vi "ConvertBoolArray4x8ToIntArray1x32.vi"(7 "boolMatrix4x8":bool[][](array[boolean])) -> (8 "intArray1x32":u32[](array[numeric]))   [LabVIEW 2016]
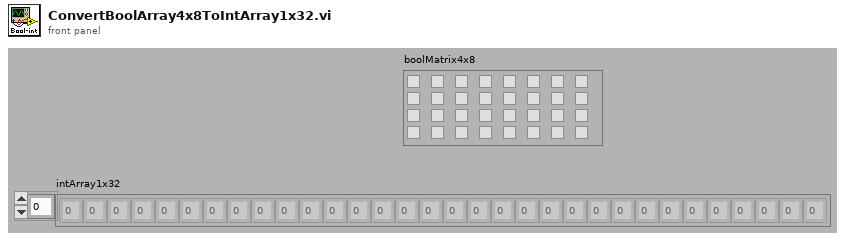
[diagram p1: front panel]
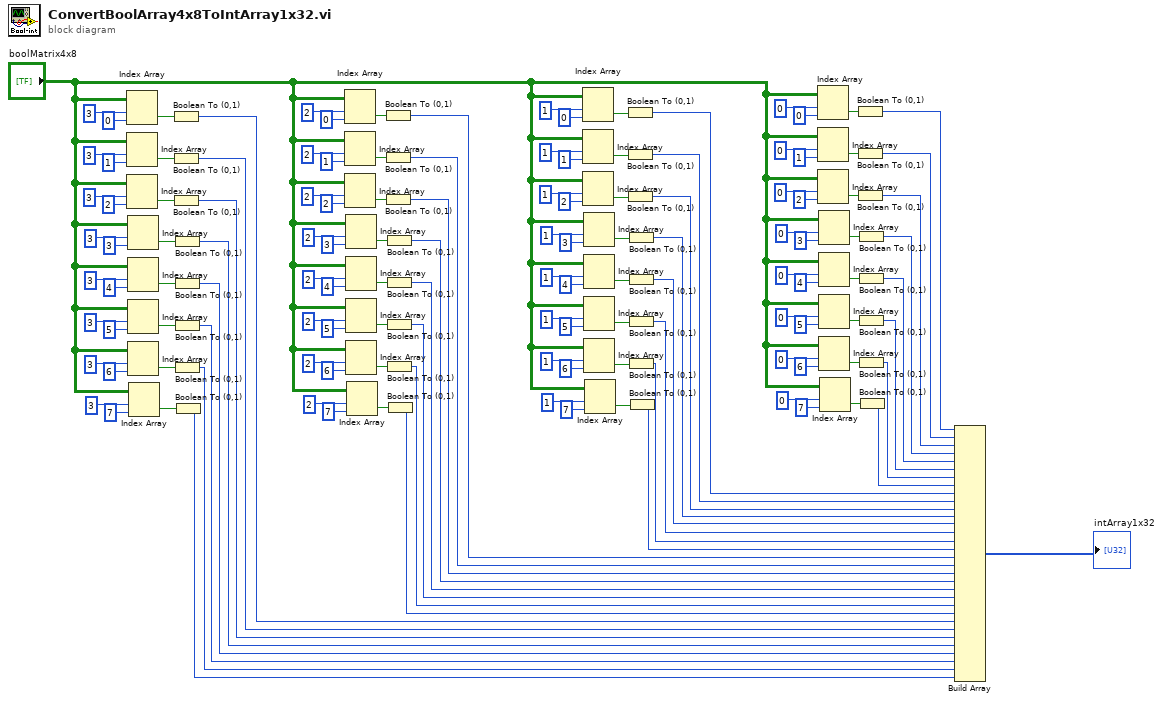
[diagram p0: block diagram]
diagram:
  n1 = Index Array(array="boolMatrix4x8", index (row)=3, index (col)=0) -> (element=w10:bool)
  n2 = Index Array(array="boolMatrix4x8", index (row)=3, index (col)=1) -> (element=w11:bool)
  n3 = Index Array(array="boolMatrix4x8", index (row)=3, index (col)=2) -> (element=w12:bool)
  n4 = Index Array(array="boolMatrix4x8", index (row)=3, index (col)=3) -> (element=w13:bool)
  n5 = Index Array(array="boolMatrix4x8", index (row)=3, index (col)=4) -> (element=w14:bool)
  n6 = Index Array(array="boolMatrix4x8", index (row)=3, index (col)=5) -> (element=w15:bool)
  n7 = Index Array(array="boolMatrix4x8", index (row)=3, index (col)=6) -> (element=w16:bool)
  n8 = Index Array(array="boolMatrix4x8", index (row)=3, index (col)=7) -> (element=w17:bool)
  n9 = Boolean To (0,1)(Boolean=w10) -> (0, 1=w9:i16)
  n10 = Boolean To (0,1)(Boolean=w11) -> (0, 1=w8:i16)
  n11 = Boolean To (0,1)(Boolean=w12) -> (0, 1=w7:i16)
  n12 = Boolean To (0,1)(Boolean=w13) -> (0, 1=w6:i16)
  n13 = Boolean To (0,1)(Boolean=w14) -> (0, 1=w5:i16)
  n14 = Boolean To (0,1)(Boolean=w15) -> (0, 1=w4:i16)
  n15 = Boolean To (0,1)(Boolean=w16) -> (0, 1=w3:i16)
  n16 = Boolean To (0,1)(Boolean=w17) -> (0, 1=w2:i16)
  n17 = Index Array(array="boolMatrix4x8", index (row)=2, index (col)=0) -> (element=w33:bool)
  n18 = Index Array(array="boolMatrix4x8", index (row)=2, index (col)=1) -> (element=w32:bool)
  n19 = Index Array(array="boolMatrix4x8", index (row)=2, index (col)=2) -> (element=w31:bool)
  n20 = Index Array(array="boolMatrix4x8", index (row)=2, index (col)=3) -> (element=w30:bool)
  n21 = Index Array(array="boolMatrix4x8", index (row)=2, index (col)=4) -> (element=w29:bool)
  n22 = Index Array(array="boolMatrix4x8", index (row)=2, index (col)=5) -> (element=w28:bool)
  n23 = Index Array(array="boolMatrix4x8", index (row)=2, index (col)=6) -> (element=w27:bool)
  n24 = Index Array(array="boolMatrix4x8", index (row)=2, index (col)=7) -> (element=w26:bool)
  n25 = Boolean To (0,1)(Boolean=w33) -> (0, 1=w25:i16)
  n26 = Boolean To (0,1)(Boolean=w32) -> (0, 1=w24:i16)
  n27 = Boolean To (0,1)(Boolean=w31) -> (0, 1=w23:i16)
  n28 = Boolean To (0,1)(Boolean=w30) -> (0, 1=w22:i16)
  n29 = Boolean To (0,1)(Boolean=w29) -> (0, 1=w21:i16)
  n30 = Boolean To (0,1)(Boolean=w28) -> (0, 1=w20:i16)
  n31 = Boolean To (0,1)(Boolean=w27) -> (0, 1=w19:i16)
  n32 = Boolean To (0,1)(Boolean=w26) -> (0, 1=w18:i16)
  n33 = Index Array(array="boolMatrix4x8", index (row)=1, index (col)=0) -> (element=w49:bool)
  n34 = Index Array(array="boolMatrix4x8", index (row)=1, index (col)=1) -> (element=w48:bool)
  n35 = Index Array(array="boolMatrix4x8", index (row)=1, index (col)=2) -> (element=w47:bool)
  n36 = Index Array(array="boolMatrix4x8", index (row)=1, index (col)=3) -> (element=w46:bool)
  n37 = Index Array(array="boolMatrix4x8", index (row)=1, index (col)=4) -> (element=w45:bool)
  n38 = Index Array(array="boolMatrix4x8", index (row)=1, index (col)=5) -> (element=w44:bool)
  n39 = Index Array(array="boolMatrix4x8", index (row)=1, index (col)=6) -> (element=w43:bool)
  n40 = Index Array(array="boolMatrix4x8", index (row)=1, index (col)=7) -> (element=w42:bool)
  n41 = Boolean To (0,1)(Boolean=w49) -> (0, 1=w39:i16)
  n42 = Boolean To (0,1)(Boolean=w48) -> (0, 1=w40:i16)
  n43 = Boolean To (0,1)(Boolean=w47) -> (0, 1=w38:i16)
  n44 = Boolean To (0,1)(Boolean=w46) -> (0, 1=w37:i16)
  n45 = Boolean To (0,1)(Boolean=w45) -> (0, 1=w36:i16)
  n46 = Boolean To (0,1)(Boolean=w44) -> (0, 1=w35:i16)
  n47 = Boolean To (0,1)(Boolean=w43) -> (0, 1=w34:i16)
  n48 = Boolean To (0,1)(Boolean=w42) -> (0, 1=w41:i16)
  n49 = Index Array(array="boolMatrix4x8", index (row)=0, index (col)=0) -> (element=w52:bool)
  n50 = Index Array(array="boolMatrix4x8", index (row)=0, index (col)=1) -> (element=w55:bool)
  n51 = Index Array(array="boolMatrix4x8", index (row)=0, index (col)=2) -> (element=w58:bool)
  n52 = Index Array(array="boolMatrix4x8", index (row)=0, index (col)=3) -> (element=w61:bool)
  n53 = Index Array(array="boolMatrix4x8", index (row)=0, index (col)=4) -> (element=w73:bool)
  n54 = Index Array(array="boolMatrix4x8", index (row)=0, index (col)=5) -> (element=w70:bool)
  n55 = Index Array(array="boolMatrix4x8", index (row)=0, index (col)=6) -> (element=w67:bool)
  n56 = Index Array(array="boolMatrix4x8", index (row)=0, index (col)=7) -> (element=w64:bool)
  n57 = Boolean To (0,1)(Boolean=w52) -> (0, 1=w75:i16)
  n58 = Boolean To (0,1)(Boolean=w55) -> (0, 1=w76:i16)
  n59 = Boolean To (0,1)(Boolean=w58) -> (0, 1=w77:i16)
  n60 = Boolean To (0,1)(Boolean=w61) -> (0, 1=w78:i16)
  n61 = Boolean To (0,1)(Boolean=w73) -> (0, 1=w79:i16)
  n62 = Boolean To (0,1)(Boolean=w70) -> (0, 1=w80:i16)
  n63 = Boolean To (0,1)(Boolean=w67) -> (0, 1=w81:i16)
  n64 = Boolean To (0,1)(Boolean=w64) -> (0, 1=w82:i16)
  n65 = Build Array(w75, w76, w77, w78, w79, w80, w81, w82, w39, w40, w38, w37, w36, w35, w34, w41, w25, w24, w23, w22, w21, w20, w19, w18, w9, w8, w7, w6, w5, w4, w3, w2) -> (→"intArray1x32":i16[])
